vi "TDMS - Fire Command.vi"(8 "error in (no error)":errorcluster, 9 "Data":variant, 10 "CMD":T1, 11 "View Model":T2) -> (0 "error out":errorcluster)   [LabVIEW 2017]
doc: "Generate TDMS command to TDMS process"
uses:
  View Model/Controls/View Model.ctl
  View Model/Controls/Shared Model.ctl
  Error Handler/Controls/Error Model.ctl
  Error Handler/Controls/Error Event.ctl
  Error Handler/Controls/Error Type.ctl
  Controller/Controls/Controller Model.ctl
  Controller/Controls/Controller Event.ctl
  Controller/Controls/Controller Command.ctl
  Controller/Controls/Controller Overhead.ctl
  Real-Time/RT Status.ctl
  Real-Time/RT Loop Status.ctl
  Controller/Controls/Controller NStream.ctl
  Controller/Controls/Controller DAQ Data.ctl
  Controls/TDMS Model.ctl
  Controls/TDMS Event.ctl
  Controls/TDMS Command.ctl
  Controls/TDMS Overhead.ctl
  Controls/TDMS ChanProperties.ctl
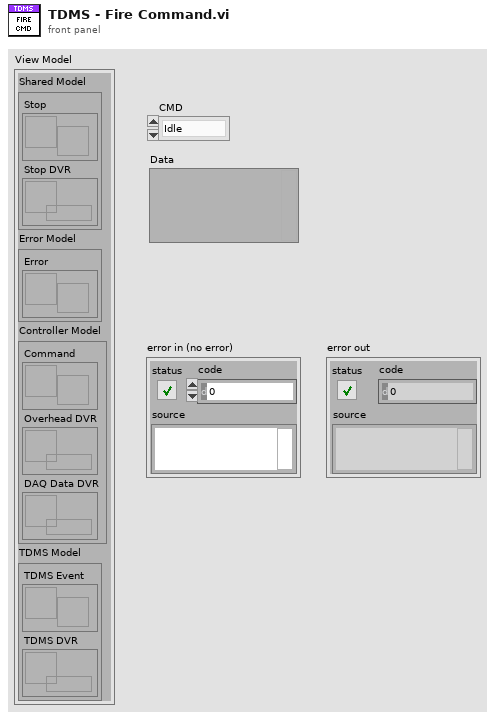
[diagram p1: front panel]
types:
  T1 = typedef "TDMS Command.ctl" = enum16{"Idle", "Create File", "Save Data", "Close Fire"}
  T2 = typedef "View Model.ctl" = cluster{"Shared Model":T3, "Error Model":T4, "Controller Model":T5, "TDMS Model":T6}
  T3 = typedef "Shared Model.ctl" = cluster{"Stop":refnum<user-event>, "Stop DVR":refnum<data-value>}
  T4 = typedef "Error Model.ctl" = cluster{"Error":refnum<user-event>}
  T5 = typedef "Controller Model.ctl" = cluster{"Command":refnum<user-event>, "Overhead DVR":refnum<data-value>, "DAQ Data DVR":refnum<data-value>}
  T6 = typedef "TDMS Model.ctl" = cluster{"TDMS Event":refnum<user-event>, "TDMS DVR":refnum<data-value>}
  T7 = typedef "TDMS Event.ctl" = cluster{"CMD":T1, "Data":variant}
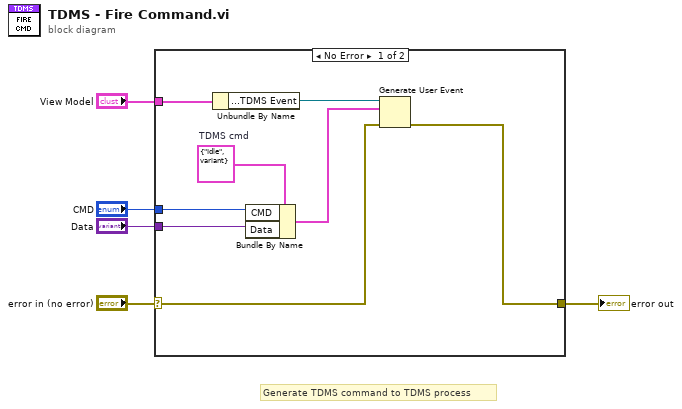
[diagram p0: block diagram]
diagram:
  # "Generate TDMS command to TDMS process"
  n1 = case shown="No Error" "error in (no error)" {
    selector: "error in (no error)" -> [w12 w14]
    tunnel: [w10 w14] -> w4
    tunnel: "View Model" -> [w11 _]
    tunnel: "Data" -> [w7 _]
    tunnel: "CMD" -> [w6 _]
    frame No Error {
      w9 = T7 {"CMD"=enum."Idle", "Data"=variant}  # TDMS cmd
      n2 = Unbundle By Name(w11) -> ("TDMS Model.TDMS Event"=w13:refnum<user-event>)
      n3 = Bundle By Name(cluster=w9, "CMD"=w6, "Data"=w7) -> (w8:T7)
      n4 = Generate User Event(user event=w13, event data cluster=w8, error in=w12) -> (error out=w10:errorcluster)  [unwired: 1 in, 1 out]
    }
    frame Error {
    }
  }
  "error out" <- w4
